vi "Obtain Bucket.vi"(8 "error in (no error)":errorcluster, 9 "Region":T1, 10 "Bucket name":string, 11 "AWS Credentials":T2) -> (0 "error out":errorcluster, 3 "Bucket":refnum<class "Bucket.lvclass">)   [LabVIEW 2018, in "NI_AWS_S3.lvlib" / "Bucket.lvclass"]
uses:
  Bucket.lvclass
  Core/HTTP Request/AWS Credentials.ctl
  C:/labview-projects/aws-toolkit/source/Core/HTTP Request/HTTP Request.lvclass
  Core/HTTP Request/Region.ctl
  Core/HTTP Request/HTTP Request.lvclass/HTTP Request.ctl
  Bucket.lvclass/Bucket.ctl
  Core/HTTP Request/Write Credentials.vi
  Core/HTTP Request/Write Region.vi
  Core/HTTP Request/Write Service.vi
  Write Name.vi
  Core/HTTP Request/HTTP Request.lvclass
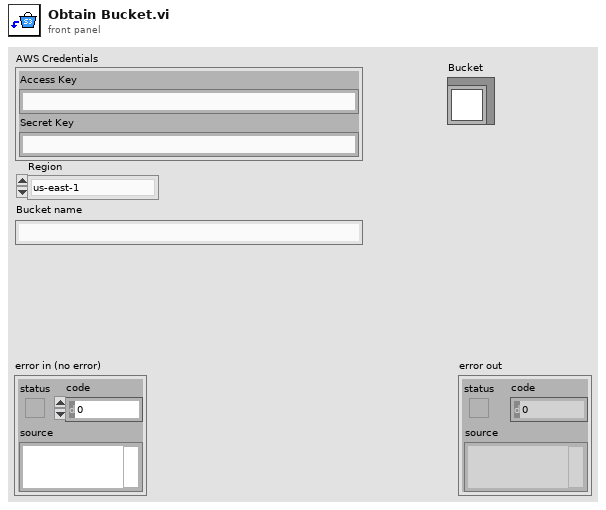
[diagram p1: front panel]
types:
  T1 = typedef "NI_AWS_Core.lvlib/HTTP Request.lvclass/Region.ctl" = enum16{"us-east-1", "us-east-2", "us-west-1", "us-west-2", "ap-northeast-1", "ap-northeast-2", "ap-southeast-1", "ap-southeast-2", "ca-central-1", "eu-central-1", "eu-west-1", "eu-west-2", "sa-east-1"}
  T2 = typedef "NI_AWS_Core.lvlib/HTTP Request.lvclass/AWS Credentials.ctl" = cluster{"Access Key":string, "Secret Key":string}
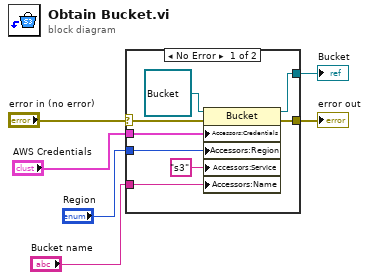
[diagram p0: block diagram]
diagram:
  n1 = case shown="No Error" "error in (no error)" {
    selector: "error in (no error)" -> [w7 w15]
    tunnel: "AWS Credentials" -> [w14 _]
    tunnel: [w13 w15] -> w5
    tunnel: [w12 _] -> w4
    tunnel: "Bucket name" -> [w11 _]
    tunnel: "Region" -> [w10 _]
    frame No Error {
      n2 = property class="Bucket"(reference=refnum<class "Bucket.lvclass"> refnum ("NI_AWS_S3.lvlib:Bucket.lvclass"), error in=w7, "Accessors:Credentials"=w14, "Accessors:Region"=w10, "Accessors:Service"="s3" ("Service"), "Accessors:Name"=w11) -> (reference out=w12:refnum<class "Bucket.lvclass">, error out=w13:errorcluster)
    }
    frame Error {
    }
  }
  "error out" <- w5
  "Bucket" <- w4
